vi "Add Routing Channel.vi"(8 "error in (no error)":errorcluster, 9 "Channel States":T1, 10 "Channel Name":string, 11 "RAF Custom Device in":refnum<k24>) -> (0 "error out":errorcluster, 2 "Channel Ref":T4 format="%.0x", 3 "RAF Custom Device out":refnum<k24>)   [LabVIEW 2017, in "Switch Scripting.lvlib"]
uses:
  Switch Scripting.lvlib
  NationalInstruments.VeriStand.SystemDefinitionAPI
  <vilib>/NI Veristand/Custom Device API/Custom Device Item Ref.ctl
  Channel States.ctl
  Routing State.ctl
  Connection.ctl
  <vilib>/NI Veristand/Custom Device API/Custom Device Channel.ctl
  <vilib>/NI Veristand/Custom Device API/Custom Device Channel Type.ctl
  <vilib>/NI Veristand/Custom Device API/Set Item Property (String).vi
  <vilib>/NI VeriStand/Custom Device API/Custom Device API.lvlib
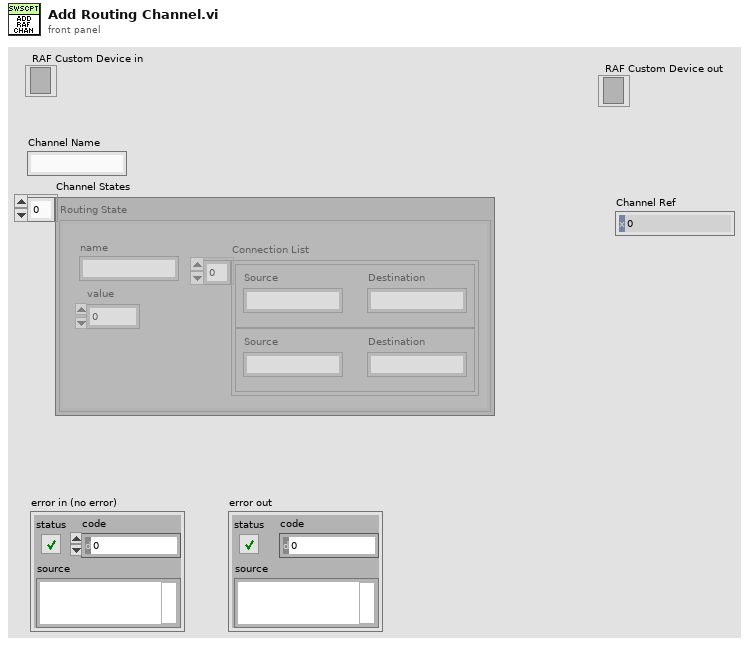
[diagram p1: front panel]
types:
  T1 = typedef "Switch Scripting.lvlib/Channel States.ctl" = T2[]
  T2 = typedef "Switch Scripting.lvlib/Routing State.ctl" = cluster{"name":string, "value":i32, "Connection List":T3[]}
  T3 = typedef "Switch Scripting.lvlib/Connection.ctl" = cluster{"Source":string, "Destination":string}
  T4 = typedef "Custom Device API.lvlib/Custom Device Item Ref.ctl" = u64
  T5 = typedef "Custom Device API.lvlib/Custom Device Channel.ctl" = cluster{"Type":T6, "Units":string, "Default Value":dbl, "Faultable":bool, "Scalable":bool}
  T6 = typedef "Custom Device API.lvlib/Custom Device Channel Type.ctl" = enum16{"Input", "Output"}
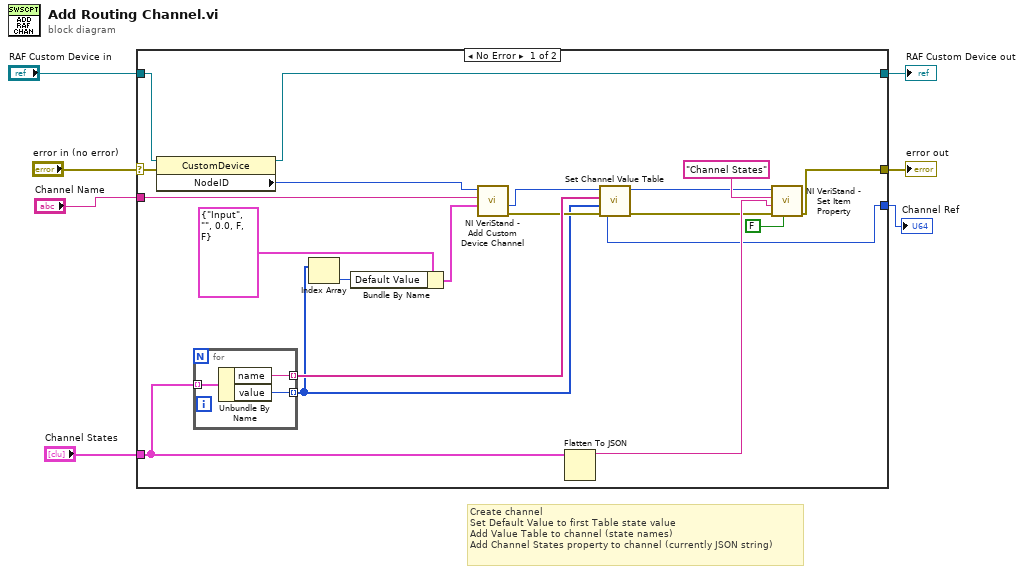
[diagram p0: block diagram]
diagram:
  # "Create channel\nSet Default Value to first Table state value\nAdd Value Table to channel (state names)\nAdd Channel States property to channel (currently JSON string)"
  n1 = case shown="No Error" "error in (no error)" {
    selector: "error in (no error)" -> [w25 w31]
    tunnel: [w20 w31] -> w7
    tunnel: [w26 w30] -> w6
    tunnel: "RAF Custom Device in" -> [w24 w30]
    tunnel: "Channel Name" -> [w22 _]
    tunnel: [w14 _] -> w2
    tunnel: "Channel States" -> [w17 _]
    frame No Error {
      n2 = property class="CustomDevice"(reference=w24, error in=w25) -> (reference out=w26:refnum<k24>, "NodeID"=w23:u64)  [unwired: 1 out]
      n3 = for {
        tunnel: w17 -> [w29] mode=indexing
        tunnel: [w28] -> w16 mode=indexing
        tunnel: [w27] -> w9 mode=indexing
        n4 = Unbundle By Name(w29) -> ("name"=w28:string, "value"=w27:i32)
      }
      n5 = Index Array(array=w9) -> (element=w8:i32)  [unwired: 1 in]
      n6 = Bundle By Name(cluster=T5 {"Type"=enum."Input", "Units"="", "Default Value"=0.0, "Faultable"=FALSE, "Scalable"=FALSE} ("Channel"), "Default Value"=w8) -> (w10:T5)
      n7 = call <vilib>:"NI VeriStand - Add Custom Device Channel.vi"("Channel"=w10, "Channel Name"=w22, "Parent Ref in"=w23) -> ("error out"=w13:errorcluster, "Channel Ref"=w15:T4)  [unwired: 5 in, 2 out]
      n8 = Flatten To JSON(anything=w17) -> (JSON string=w18:string)  [unwired: 2 in, 1 out]
      n9 = call "Set Channel Value Table.vi"("error in (no error)"=w13, "Values"=w9, "Names"=w16, "Channel Ref in"=w15) -> ("error out"=w12:errorcluster, "Channel Ref out"=w14:T4)  [unwired: 6 in]
      n10 = call-poly <vilib>:"NI VeriStand - Set Item Property.vi"("Binary String (T)"=FALSE, "error in (no error)"=w12, "Value"=w18, "Property Name"="Channel States" ("String"), "Item Ref in"=w15) -> ("error out"=w20:errorcluster)  [unwired: 4 in, 2 out]
    }
    frame Error {
    }
  }
  "error out" <- w7
  "RAF Custom Device out" <- w6
  "Channel Ref" <- w2
